vi "Create.vi"(7 "Expected Number of Calls":u32, 8 "error in (no error)":errorcluster, 10 "Comparator":refnum<class "Comparator.lvclass">) -> (0 "error out":errorcluster, 3 "Exactly Out":refnum<class "Exactly.lvclass">)   [LabVIEW 2020, in "Deprecated Exactly.lvlib" / "Exactly.lvclass"]
uses:
  Exactly.lvclass
  Core/Comparator/Comparator.lvclass
  Exactly.lvclass/Exactly.ctl
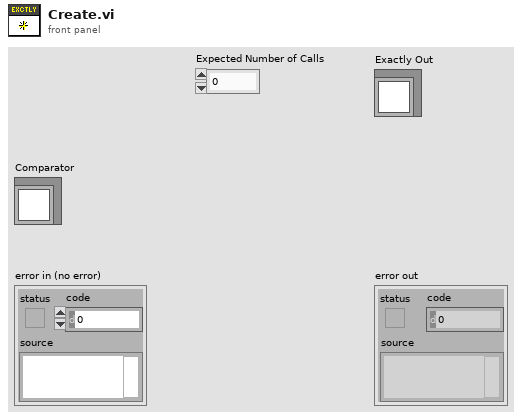
[diagram p1: front panel]
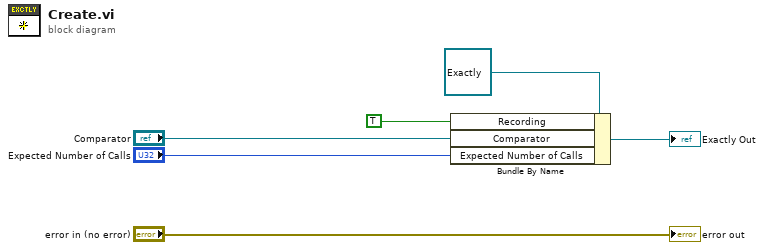
[diagram p0: block diagram]
diagram:
  n1 = Bundle By Name(cluster=refnum<class "Exactly.lvclass"> refnum ("One"), "Recording"=TRUE, "Comparator"="Comparator", "Expected Number of Calls"="Expected Number of Calls") -> (→"Exactly Out":refnum<class "Exactly.lvclass">)
  "error out" <- "error in (no error)"
